vi "SDCP BTR Encode.vi"(4 "error in (no error)":errorcluster, 7 "in":T1) -> (0 "error out":errorcluster, 1 "BTR3 encoded":u8[](array[numeric]), 2 "BTR2 encoded":u8[](array[numeric]), 3 "BTR1 encoded":u8[](array[numeric]))   [LabVIEW 2020]
uses:
  Typedefs/SDCP BTR Params.ctl
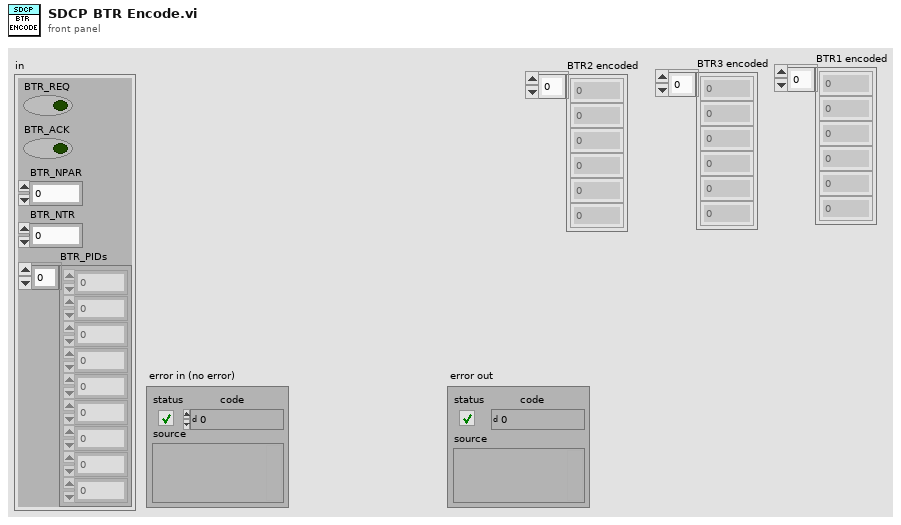
[diagram p1: front panel]
types:
  T1 = typedef "SDCP BTR Params.ctl" = cluster{"BTR_REQ":bool, "BTR_ACK":bool, "BTR_NPAR":i32, "BTR_NTR":i32, "BTR_PIDs":u8[]}
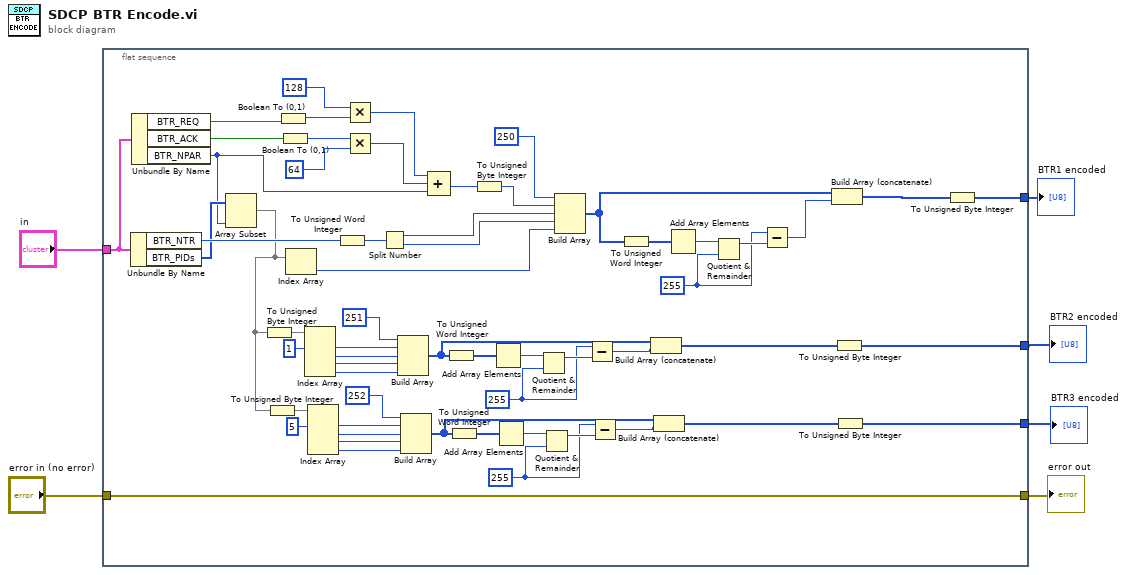
[diagram p0: block diagram]
diagram:
  n1 = flat-sequence {
    tunnel: "in" -> [w14]
    tunnel: [w9] -> w1
    tunnel: "error in (no error)" -> [w42]
    tunnel: [w42] -> w4
    tunnel: [w8] -> w3
    tunnel: [w7] -> w2
    frame #0 {
      w18 = u16 255 ("y")
      w32 = u16 255 ("y")
      w47 = u16 255 ("y")
      n2 = Unbundle By Name(w14) -> ("BTR_NTR"=w13:i32, "BTR_PIDs"=w12:u8[])
      n3 = Unbundle By Name(w14) -> ("BTR_REQ"=w65:bool, "BTR_ACK"=w64:bool, "BTR_NPAR"=w11:i32)
      n4 = Array Subset(array=w12, length=w11) -> (w10:u8[])  [unwired: 1 in]
      n5 = To Unsigned Byte Integer(number=w10) -> (unsigned 8bit integer=w41:u8[])
      n6 = To Unsigned Byte Integer(number=w10) -> (unsigned 8bit integer=w27:u8[])
      n7 = Boolean To (0,1)(Boolean=w65) -> (0, 1=w63:i16)
      n8 = Boolean To (0,1)(Boolean=w64) -> (0, 1=w61:i16)
      n9 = Index Array(array=w10) -> (element=w51:u8)  [unwired: 1 in]
      n10 = Index Array(array=w41, index #1=1 ("index")) -> (element #1=w40:u8, element #2=w39:u8, element #3=w38:u8, element #4=w37:u8)  [unwired: 3 in]
      n11 = Index Array(array=w27, index #1=5 ("index")) -> (element #1=w26:u8, element #2=w25:u8, element #3=w24:u8, element #4=w23:u8)  [unwired: 3 in]
      n12 = To Unsigned Word Integer(number=w13) -> (unsigned 16bit integer=w57:u16)
      n13 = Multiply(x=i16 128, y=w63) -> (x*y=w59:i16)
      n14 = Multiply(x=w61, y=i16 64) -> (x*y=w58:i16)
      n15 = Split Number(x=w57) -> (hi(x)=w54:u8, lo(x)=w53:u8)
      n16 = Build Array(u8 251 ("element"), w40, w39, w38, w37) -> (w30:u8[])
      n17 = Build Array(u8 252 ("element"), w26, w25, w24, w23) -> (w16:u8[])
      n18 = Compound Arithmetic op=ADD(w59, w58, w11) -> (w55:i32)
      n19 = To Unsigned Word Integer(number=w30) -> (unsigned 16bit integer=w35:u16[])
      n20 = To Unsigned Word Integer(number=w16) -> (unsigned 16bit integer=w21:u16[])
      n21 = To Unsigned Byte Integer(number=w55) -> (unsigned 8bit integer=w56:u8)
      n22 = Add Array Elements(numeric array=w35) -> (sum=w34:u16)
      n23 = Add Array Elements(numeric array=w21) -> (sum=w20:u16)
      n24 = Quotient & Remainder(x=w34, y=w32) -> (x-y*floor(x/y)=w33:u16)  [unwired: 1 out]
      n25 = Quotient & Remainder(x=w20, y=w18) -> (x-y*floor(x/y)=w19:u16)  [unwired: 1 out]
      n26 = Build Array(u8 250 ("element"), w56, w54, w53, w51) -> (w46:u8[])
      n27 = Subtract(x=w32, y=w33) -> (x-y=w31:u16)
      n28 = Subtract(x=w18, y=w19) -> (x-y=w17:u16)
      n29 = To Unsigned Word Integer(number=w46) -> (unsigned 16bit integer=w50:u16[])
      n30 = Build Array (concatenate)(w30, w31) -> (w29:u16[])
      n31 = Build Array (concatenate)(w16, w17) -> (w15:u16[])
      n32 = Add Array Elements(numeric array=w50) -> (sum=w49:u16)
      n33 = Quotient & Remainder(x=w49, y=w47) -> (x-y*floor(x/y)=w48:u16)  [unwired: 1 out]
      n34 = Subtract(x=w47, y=w48) -> (x-y=w45:u16)
      n35 = Build Array (concatenate)(w46, w45) -> (w44:u16[])
      n36 = To Unsigned Byte Integer(number=w29) -> (unsigned 8bit integer=w8:u8[])
      n37 = To Unsigned Byte Integer(number=w15) -> (unsigned 8bit integer=w7:u8[])
      n38 = To Unsigned Byte Integer(number=w44) -> (unsigned 8bit integer=w9:u8[])
    }
  }
  "error out" <- w4
  "BTR2 encoded" <- w3
  "BTR3 encoded" <- w2
  "BTR1 encoded" <- w1
